vi "Assert Session Count.vi"(8 "error in":errorcluster, 10 "expected value":i32, 11 "session reservation in":refnum<class "Session Reservation.lvclass">) -> (0 "error out":errorcluster, 1 "result":string, 2 "pass":bool, 3 "session reservation out":refnum<class "Session Reservation.lvclass">)   [LabVIEW 2020, in "MeasurementServerTests.lvlib" / "Session Reservation Tests.lvlib"]
uses:
  Session Reservation Tests.lvlib
  Runtime/MeasurementLink Session Management/Session Reservation/Session Reservation.lvclass
  Runtime/MeasurementLink Session Management/Session Reservation/Get Session Info - NSess .vi
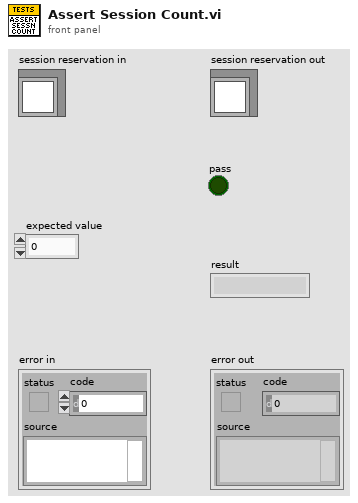
[diagram p1: front panel]
types:
  T1 = typedef "MeasurementLink Session Management Client.lvlib/ni_measurementlink_sessionmanagement_v1_SessionInformation.ctl" = cluster{"session":T2, "resource_name":string, "channel_list":string, "instrument_type_id":string, "session_exists":bool, "channel_mappings":T3[]}
  T2 = typedef "MeasurementLink Session Management Client.lvlib/nidevice_grpc_Session.ctl" = cluster{"name":string}
  T3 = typedef "MeasurementLink Session Management Client.lvlib/ni_measurementlink_sessionmanagement_v1_ChannelMapping.ctl" = cluster{"pin_or_relay_name":string, "site":i32, "channel":string}
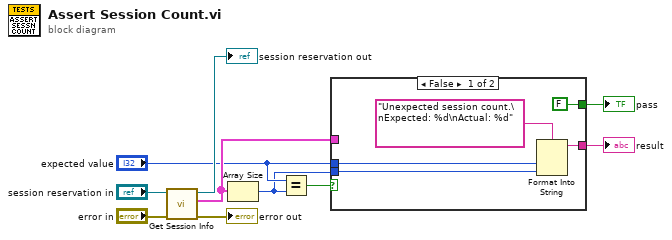
[diagram p0: block diagram]
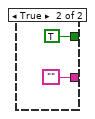
[diagram p2: hidden frame]
diagram:
  n1 = call-poly "Get Session Info.vi"("error in"="error in", "session reservation in"="session reservation in") -> ("error out"=→"error out":errorcluster, "sessions info"=w4:T1[], "session reservation out"=→"session reservation out":refnum<class "Session Reservation.lvclass">)  [unwired: 7 in]
  n2 = Array Size(array=w4) -> (size(s)=w1:i32)
  n3 = Equal?(x="expected value", y=w1) -> (x = y?=w3:bool)
  n4 = case shown="False" w3 {
    tunnel: [FALSE ("pass") TRUE ("pass")] -> w6
    tunnel: [w13 ""] -> w5
    tunnel: w4 -> [_ _]
    tunnel: "expected value" -> [w12 _]
    tunnel: w1 -> [w11 _]
    frame False {
      n5 = Format Into String(format string="Unexpected session count.\nExpected: %d\nActual: %d", w12, w11) -> (resulting string=w13:string)  [unwired: 2 in, 1 out]
    }
    frame True {
    }
  }
  "pass" <- w6
  "result" <- w5
